vi "Get DAQmx AI Task Ref from AI TaskName.vi"(8 "error in (no error)":errorcluster, 10 "AI TaskName":string, 11 "DAQ":refnum<class "DAQ.lvclass">) -> (0 "error out":errorcluster, 2 "DAQmx AI Task":refnum<k21>, 3 "DAQ":refnum<class "DAQ.lvclass">)   [LabVIEW 2017, in "DAQ.lvclass"]
doc: "Developed by Kevin Thompson\nkevin@thompsonengineering.net\n\nCopyright 2018-2020\nThompson Engineering, LLC"
uses:
  DAQ.lvclass
  DAQ.lvclass/DAQ.ctl
  DataTypes/TD AI TaskIO.ctl
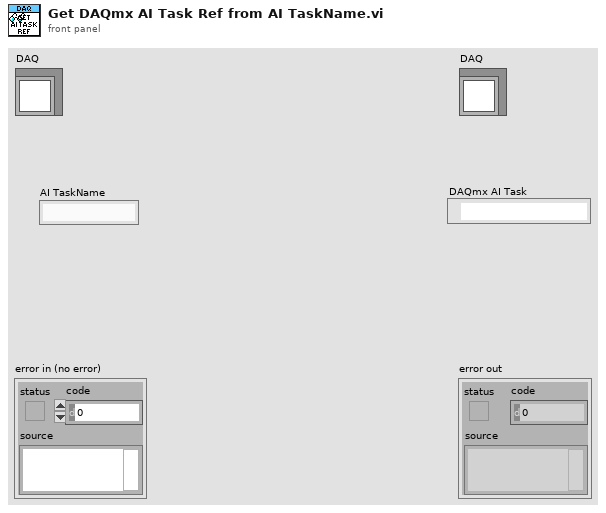
[diagram p1: front panel]
types:
  T1 = typedef "DAQ.lvclass/TD AI TaskIO.ctl" = cluster{"AI TaskName":string, "IONames":string[], "DAQmx AI TaskRef":refnum<k21>}
  T2 = typedef "TD Dynamic CVT DVR--ref.ctl" = refnum<data-value>
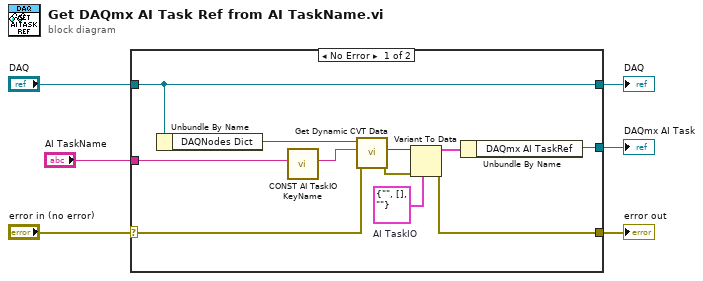
[diagram p0: block diagram]
diagram:
  n1 = case shown="No Error" "error in (no error)" {
    selector: "error in (no error)" -> [w15 w18]
    tunnel: [w14 w18] -> w5
    tunnel: [w17 w19] -> w3
    tunnel: "DAQ" -> [w17 w19]
    tunnel: "AI TaskName" -> [w11 _]
    tunnel: [w7 _] -> w1
    frame No Error {
      w9 = T1 {"AI TaskName"="", "IONames"=[], "DAQmx AI TaskRef"=""}  # AI TaskIO
      n2 = Unbundle By Name(w17) -> ("DAQNodes Dict"=w16:T2)
      n3 = call "CONST AI TaskIO KeyName.vi"("AI TaskName"=w11) -> ("AI TaskIO (KeyName)"=w10:string)  [unwired: 10 in]
      n4 = call <vilib>:"Get Dynamic CVT Data.vi"("error in (no error)"=w15, "DataName"=w10, "dCVT DVR"=w16) -> ("error out"=w13:errorcluster, "value"=w12:variant)  [unwired: 5 in, 2 out]
      n5 = Variant To Data(error in=w13, type=w9, Variant=w12) -> (data=w8:T1, error out=w14:errorcluster)
      n6 = Unbundle By Name(w8) -> ("DAQmx AI TaskRef"=w7:refnum<k21>)
    }
    frame Error {
    }
  }
  "error out" <- w5
  "DAQ" <- w3
  "DAQmx AI Task" <- w1
